vi "PH_TKTDS-30xx.Evt Call Set Trigger Configuration.vi"(0 "i ref in":refnum<vi>, 1 "Instance":string="N/A", 2 "Trigger Configuration":T1={"Source"="CH1", "Slope"=0, "Level [V]"=0.0} {"Level [V]" format="%#_6p"}, 5 "error in (no error)":errorcluster) -> (14 "i ref out":refnum<vi>, 19 "error out":errorcluster)   [LabVIEW 2014, in "PH_TKTDS-30xx.lvlib"]
doc: "This VI calls sets a simple call."
uses:
  PH_TKTDS-30xx.lvlib
  PH_TKTDS-30xx.Trigger Config.ctl
  CSCore/CSSystem/CoreLib/CoreLib.double 2 byte array.vi
  CSCore/CSSystem/CoreLib/CoreLib.int 2 byte array.vi
  CSCore/CSSystem/CoreLib/CoreLib.string 2 byte array.vi
  CSCore/CSSystem/CoreLib/CoreLib.lvlib
  CSCore/BaseProcess/BaseProcess.lvlib
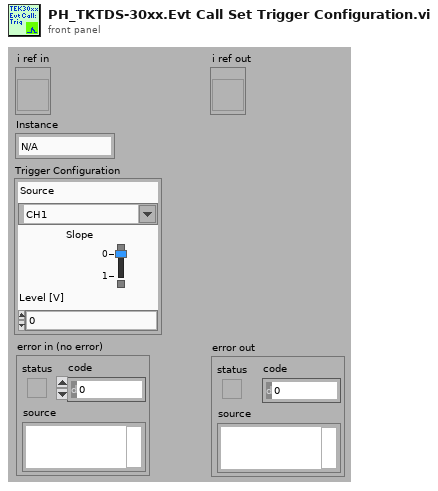
[diagram p1: front panel]
types:
  T1 = typedef "PH_TKTDS-30xx.lvlib/PH_TKTDS-30xx.Trigger Config.ctl" = cluster{"Source":string, "Slope":i32, "Level [V]":dbl}
  T2 = typedef "CoreDefs.rawDataType.ctl" = i8[]
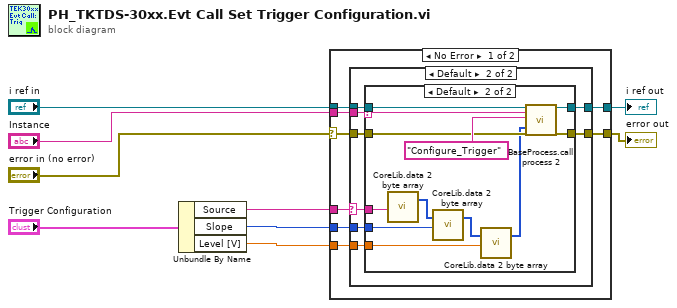
[diagram p0: block diagram]
diagram:
  n1 = Unbundle By Name("Trigger Configuration") -> ("Source"=w3:string, "Slope"=w2:i32, "Level [V]"=w1:dbl)
  n2 = case shown="No Error" "error in (no error)" {
    selector: "error in (no error)" -> [w13 w42]
    tunnel: [w17 w43] -> w9
    tunnel: [w16 w42] -> w8
    tunnel: "i ref in" -> [w15 w43]
    tunnel: w3 -> [w12 _]
    tunnel: "Instance" -> [w14 _]
    tunnel: w2 -> [w11 _]
    tunnel: w1 -> [w10 _]
    frame No Error {
      n3 = case shown="Default" w12 {
        selector: w12 -> [_ w22]
        tunnel: [w19 w27] -> w17
        tunnel: [w18 w26] -> w16
        tunnel: w15 -> [w19 w25]
        tunnel: w14 -> [_ w24]
        tunnel: w13 -> [w18 w23]
        tunnel: w11 -> [_ w21]
        tunnel: w10 -> [_ w20]
        frame "", "N/A" {
        }
        frame Default {
          n4 = case shown="Default" w24 {
            selector: w24 -> [_ w36]
            tunnel: [w28 w40] -> w27
            tunnel: [w29 w39] -> w26
            tunnel: w25 -> [w28 w38]
            tunnel: w23 -> [w29 w37]
            tunnel: w22 -> [_ w35]
            tunnel: w21 -> [_ w34]
            tunnel: w20 -> [_ w32]
            frame "N/A" {
            }
            frame Default {
              n5 = call-poly "CoreLib.data 2 byte array.vi"("string"=w35) -> ("byteArray out"=w33:T2)  [unwired: 18 in]
              n6 = call-poly "CoreLib.data 2 byte array.vi"("byteArray"=w33, "i32"=w34) -> ("byteArray out"=w31:T2)  [unwired: 17 in]
              n7 = call-poly "CoreLib.data 2 byte array.vi"("byteArray"=w31, "f64"=w32) -> ("byteArray out"=w30:T2)  [unwired: 17 in]
              n8 = call "BaseProcess.call process 2.vi"("i ref in"=w38, "Object"=w36, "Selector"="Configure_Trigger", "Data"=w30, "error in (no error)"=w37) -> ("i ref out"=w40:refnum<vi>, "error out"=w39:errorcluster)  [unwired: 13 in]
            }
          }
        }
      }
    }
    frame Error {
    }
  }
  "i ref out" <- w9
  "error out" <- w8
